vi "Polynomial Equation.vi"(8 "Y-Int":dbl, 9 "Slope":dbl, 10 "X^2 Coeff.":dbl, 11 "X":dbl) -> (3 "Output":dbl)   [LabVIEW 2020]
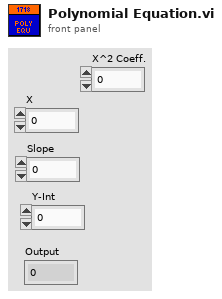
[diagram p1: front panel]
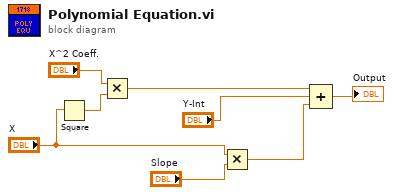
[diagram p0: block diagram]
diagram:
  n1 = Square(x="X") -> (x^2=w6:dbl)
  n2 = Multiply(x="X^2 Coeff.", y=w6) -> (x*y=w4:dbl)
  n3 = Multiply(x="X", y="Slope") -> (x*y=w2:dbl)
  n4 = Compound Arithmetic op=ADD(w4, "Y-Int", w2) -> (→"Output":dbl)
